vi "Pre Launch Init.vi"(11 "Actor_Controller_Template in":refnum<class "Actor_Controller_Template.lvclass">) -> (0 "error out":errorcluster, 3 "Actor_Controller_Template out":refnum<class "Actor_Controller_Template.lvclass">)   [LabVIEW 2020, in "Actor_Controller_Template.lvlib" / "Actor_Controller_Template.lvclass"]
doc: "(<B>Filename</B>: Actor Framework.lvlib:Actor.lvclass:Pre Launch Init.vi)\n\nDefines behavior that occurs after the Launch Nested Actor method is invoked but before the actor's Actor Core method begins running.\n\nBy default, this method does nothing. A descendant class may override it to define behavior."
uses:
  Actor_Controller_Template.lvclass
  <vilib>/ActorFramework/Actor/Actor.lvclass
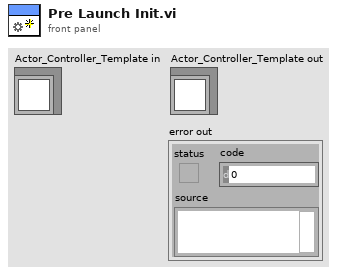
[diagram p1: front panel]
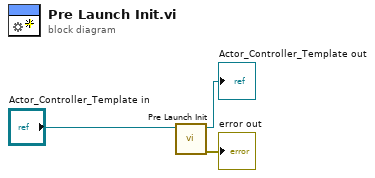
[diagram p0: block diagram]
diagram:
  n1 = call-parent "Pre Launch Init.vi"("Actor in"="Actor_Controller_Template in") -> ("error out"=→"error out":errorcluster, "Actor out"=→"Actor_Controller_Template out":refnum<class "Actor_Controller_Template.lvclass">)  [unwired: 9 in]
